vi "ReadXBOX_Control_Reference.vi"(8 "error in (no error)":errorcluster caption="错误输入（无错误）", 11 "CoordinatorState输入":refnum<class "CoordinatorState.lvclass">) -> (0 "error out":errorcluster caption="错误输出", 2 "XBOX_Control_Reference":refnum<vi>, 3 "CoordinatorState输出":refnum<class "CoordinatorState.lvclass">)   [LabVIEW 2014, in "States.lvlib" / "CoordinatorState.lvclass"]
uses:
  CoordinatorState.lvclass
  CoordinatorState.lvclass/CoordinatorState.ctl
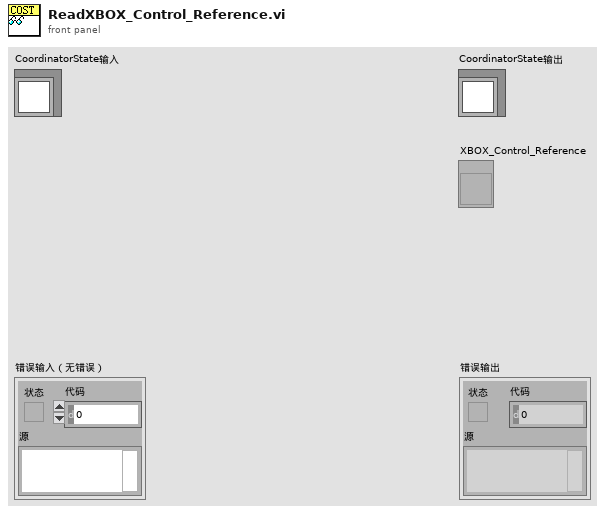
[diagram p1: front panel]
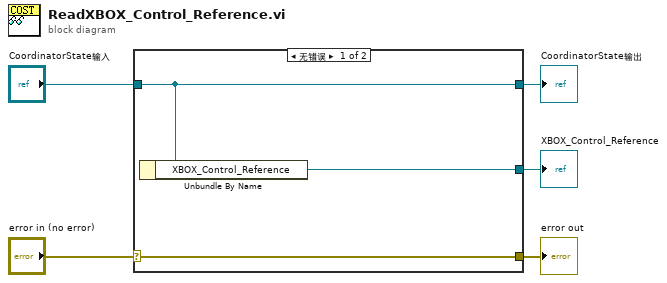
[diagram p0: block diagram]
diagram:
  n1 = case shown="无错误" "error in (no error)" {
    selector: "error in (no error)" -> [w8 w9]
    tunnel: [w8 w9] -> w4
    tunnel: [w7 w10] -> w2
    tunnel: "CoordinatorState输入" -> [w7 w10]
    tunnel: [w6 _] -> w1
    frame No Error {
      n2 = Unbundle By Name(w7) -> ("XBOX_Control_Reference"=w6:refnum<vi>)
    }
    frame Error {
    }
  }
  "error out" <- w4
  "CoordinatorState输出" <- w2
  "XBOX_Control_Reference" <- w1
